vi "Grafica.vi"(0 "ERD Data Out out":T1[](array[typedef]) {"ERD Number" format="%.0x"}) -> (8 "Graph":cluster{u32, u32, u32, u32, u32, u32}(graph))   [LabVIEW 2023]
uses:
  Common/LabVIEW GEA2 Toolkit/GEA3/type defs/ERD Read Data Out.ctl
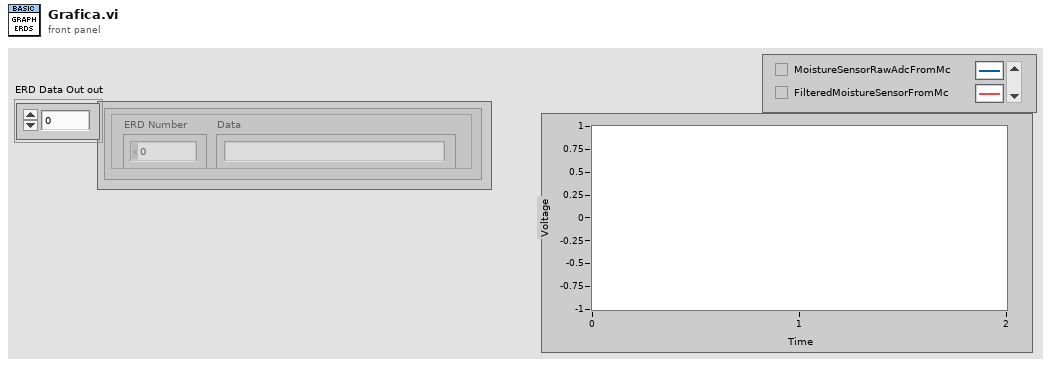
[diagram p1: front panel]
types:
  T1 = typedef "ERD Read Data Out.ctl" = cluster{"ERD Number":u16, "Data":string}
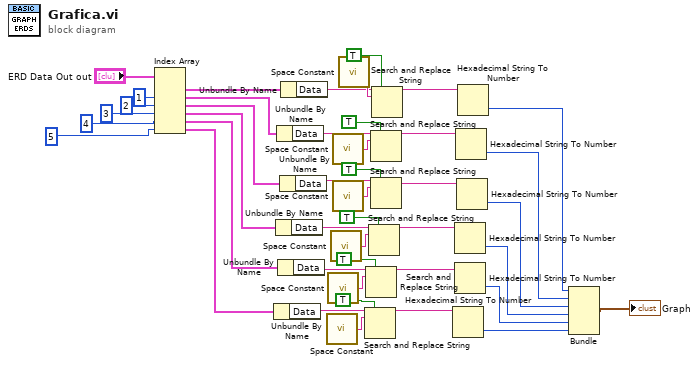
[diagram p0: block diagram]
diagram:
  n1 = Index Array(array="ERD Data Out out", index #2=1 ("index"), index #3=2 ("index"), index #4=3 ("index"), index #5=4 ("index"), index #6=5 ("index")) -> (element #1=w42:T1, element #2=w41:T1, element #3=w35:T1, element #4=w34:T1, element #5=w33:T1, element #6=w32:T1)  [unwired: 1 in]
  n2 = Unbundle By Name(w32) -> ("Data"=w3:string)
  n3 = Unbundle By Name(w34) -> ("Data"=w11:string)
  n4 = Unbundle By Name(w41) -> ("Data"=w17:string)
  n5 = Unbundle By Name(w33) -> ("Data"=w6:string)
  n6 = Unbundle By Name(w35) -> ("Data"=w14:string)
  n7 = Unbundle By Name(w42) -> ("Data"=w22:string)
  n8 = call <vilib>:"Space Constant.vi"() -> ("String"=w4:string)
  n9 = call <vilib>:"Space Constant.vi"() -> ("String"=w7:string)
  n10 = call <vilib>:"Space Constant.vi"() -> ("String"=w12:string)
  n11 = call <vilib>:"Space Constant.vi"() -> ("String"=w20:string)
  n12 = call <vilib>:"Space Constant.vi"() -> ("String"=w16:string)
  n13 = call <vilib>:"Space Constant.vi"() -> ("String"=w23:string)
  n14 = Search and Replace String(replace all?=TRUE ("replace all? (F)"), input string=w3, search string=w4) -> (result string=w1:string)  [unwired: 5 in, 3 out]
  n15 = Search and Replace String(replace all?=TRUE ("replace all? (F)"), input string=w6, search string=w7) -> (result string=w5:string)  [unwired: 5 in, 3 out]
  n16 = Search and Replace String(replace all?=TRUE ("replace all? (F)"), input string=w11, search string=w12) -> (result string=w10:string)  [unwired: 5 in, 3 out]
  n17 = Search and Replace String(replace all?=TRUE ("replace all? (F)"), input string=w17, search string=w20) -> (result string=w18:string)  [unwired: 5 in, 3 out]
  n18 = Search and Replace String(replace all?=TRUE ("replace all? (F)"), input string=w14, search string=w16) -> (result string=w15:string)  [unwired: 5 in, 3 out]
  n19 = Search and Replace String(replace all?=TRUE ("replace all? (F)"), input string=w22, search string=w23) -> (result string=w21:string)  [unwired: 5 in, 3 out]
  n20 = Hexadecimal String To Number(string=w1) -> (number=w31:u32)  [unwired: 2 in, 1 out]
  n21 = Hexadecimal String To Number(string=w10) -> (number=w29:u32)  [unwired: 2 in, 1 out]
  n22 = Hexadecimal String To Number(string=w5) -> (number=w30:u32)  [unwired: 2 in, 1 out]
  n23 = Hexadecimal String To Number(string=w18) -> (number=w27:u32)  [unwired: 2 in, 1 out]
  n24 = Hexadecimal String To Number(string=w15) -> (number=w28:u32)  [unwired: 2 in, 1 out]
  n25 = Hexadecimal String To Number(string=w21) -> (number=w26:u32)  [unwired: 2 in, 1 out]
  n26 = Bundle(w26, w27, w28, w29, w30, w31) -> (→"Graph":cluster{u32, u32, u32, u32, u32, u32})  [unwired: 1 in]
